vi "SetPWMFreq.vi"(8 "error in (no error)":errorcluster, 10 "Freq":sgl, 11 "PCA in":refnum<class "PCA.lvclass">) -> (0 "error out":errorcluster, 3 "PCA out":refnum<class "PCA.lvclass">)   [LabVIEW 2022 SP3, in "PCA9685.lvlib" / "PCA.lvclass"]
uses:
  PCA.lvclass
  PCA.lvclass/PCA.ctl
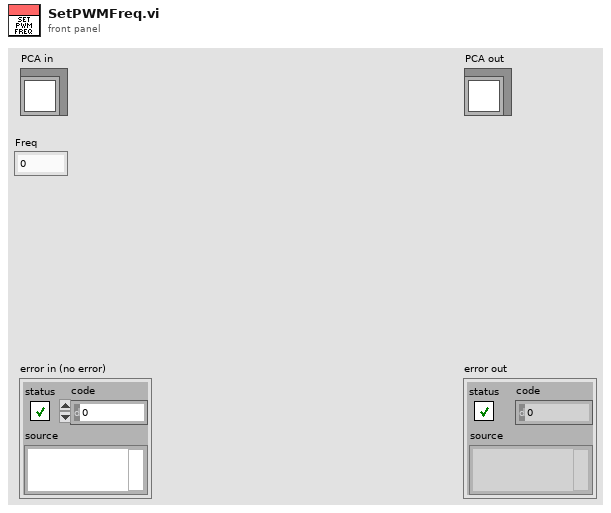
[diagram p1: front panel]
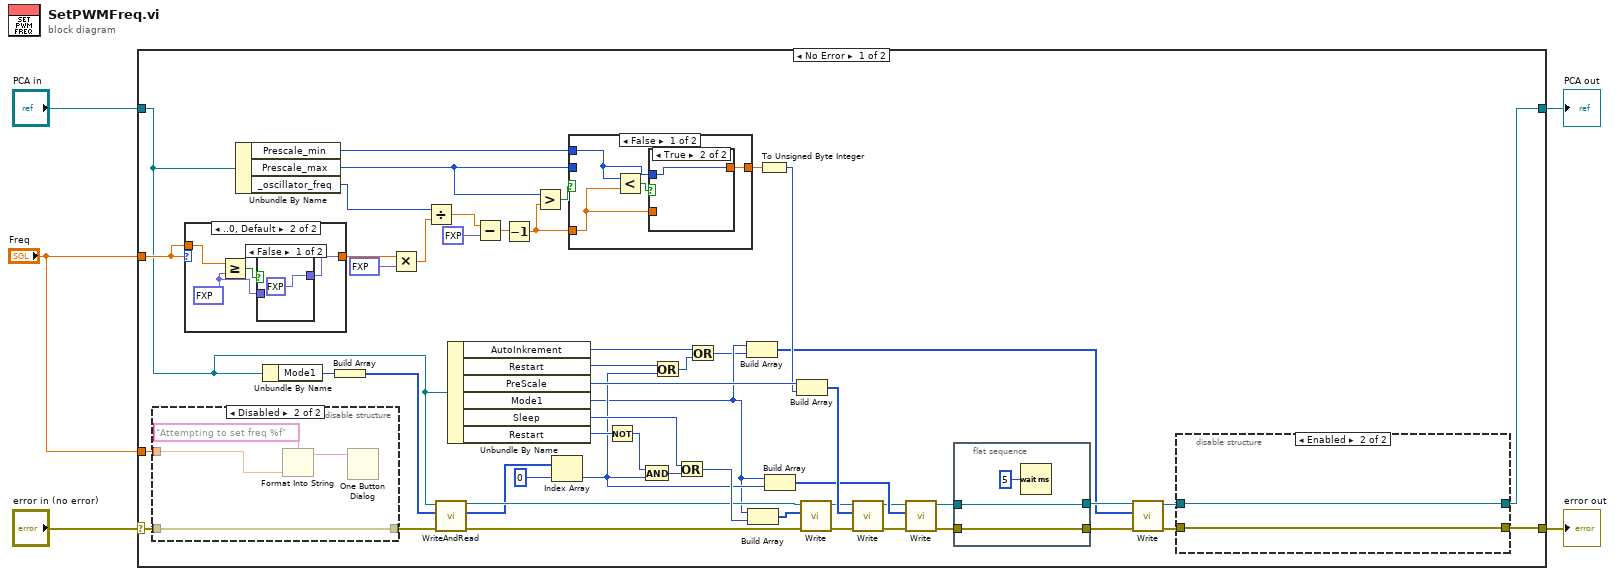
[diagram p0: block diagram]
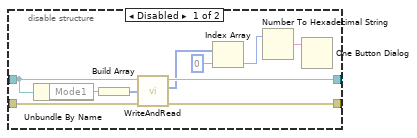
[diagram p2: hidden frame]
diagram:
  n1 = case shown="No Error" "error in (no error)" {
    selector: "error in (no error)" -> [w57 w93]
    tunnel: [w7 w93] -> w4
    tunnel: [w6 w92] -> w2
    tunnel: "PCA in" -> [w27 w92]
    tunnel: "Freq" -> [w56 _]
    tunnel: "Freq" -> [w55 _]
    frame No Error {
      n2 = disable-structure shown="Disabled" {
        disable-tunnel: w57 -> [w73 w77]
        disable-tunnel: [w73 w77] -> w54
        disable-tunnel: w56 -> [_ w76]
        frame Enabled {
        }
        frame Disabled {
          n3 = Format Into String(format string="Attempting to set freq %f", w76) -> (resulting string=w74:string)  [unwired: 2 in, 1 out]
          n4 = One Button Dialog(message=w74) -> ()  [unwired: 1 in, 1 out]
        }
      }
      n5 = case shown="..0, Default" w55 {
        tunnel: [w85 w89] -> w53
        tunnel: w55 -> [w85 w88]
        frame 1..3500 {
        }
        frame ..0, Default {
          w86 = fxp<+/-,64,32> 3500.0 ("y")
          n6 = Greater Or Equal?(x=w88, y=w86) -> (x >= y?=w87:bool)
          n7 = case shown="False" w87 {
            tunnel: [fxp<+/-,64,32> 1.0 ("Numeric") w91] -> w89
            tunnel: w86 -> [_ w91]
            frame False {
            }
            frame True {
            }
          }
        }
      }
      n8 = Unbundle By Name(w27) -> ("Prescale_min"=w43:u32, "Prescale_max"=w45:u32, "_oscillator_freq"=w50:u32)
      n9 = Unbundle By Name(w27) -> ("Mode1"=w42:u8)
      n10 = Build Array(w42) -> (w41:u8[])
      n11 = Multiply(x=w53, y=fxp<+/-,64,32> 4096.0) -> (x*y=w51:sgl)
      n12 = Divide(x=w50, y=w51) -> (x/y=w49:sgl)
      n13 = call "WriteAndRead.vi"("error in (no error)"=w54, "Data"=w41, "PCA in"=w27) -> ("error out"=w26:errorcluster, "Data 2"=w24:u8[], "PCA out"=w25:refnum<class "PCA.lvclass">)  [unwired: 6 in]
      n14 = Unbundle By Name(w27) -> ("AutoInkrement"=w16:u8, "Restart"=w18:u8, "PreScale"=w30:u8, "Mode1"=w11:u8, "Sleep"=w37:u8, "Restart"=w39:u8)
      n15 = Subtract(x=w49, y=fxp<+/-,64,33> 0.5) -> (x-y=w47:sgl)
      n16 = Decrement(x=w47) -> (x-1=w44:sgl)
      n17 = Greater?(x=w45, y=w44) -> (0:w46:bool)
      n18 = Index Array(array=w24, index=0) -> (element=w13:u8)
      n19 = case shown="False" w46 {
        tunnel: [w79 w84] -> w29
        tunnel: w45 -> [_ w84]
        tunnel: w44 -> [w78 _]
        tunnel: w43 -> [w80 _]
        frame False {
          n20 = Less?(x=w80, y=w78) -> (x < y?=w81:bool)
          n21 = case shown="True" w81 {
            tunnel: w80 -> [_ w83]
            tunnel: [w82 w83] -> w79
            tunnel: w78 -> [w82 _]
            frame False {
            }
            frame True {
            }
          }
        }
        frame True {
        }
      }
      n22 = Not(x=w39) -> (.not. x?=w38:u8)
      n23 = And(x=w38, y=w13) -> (x .and. y?=w40:u8)
      n24 = Or(x=w18, y=w13) -> (x .or. y?=w17:u8)
      n25 = Or(x=w37, y=w40) -> (x .or. y?=w35:u8)
      n26 = Or(x=w16, y=w17) -> (x .or. y?=w10:u8)
      n27 = Build Array(w11, w10) -> (w12:u8[])
      n28 = Build Array(w11, w35) -> (w34:u8[])
      n29 = To Unsigned Byte Integer(number=w29) -> (unsigned 8bit integer=w28:u8)
      n30 = Build Array(w11, w13) -> (w22:u8[])
      n31 = Build Array(w30, w28) -> (w33:u8[])
      n32 = call "Write.vi"("error in (no error)"=w26, "Data"=w34, "PCA in"=w25) -> ("error out"=w32:errorcluster, "PCA out"=w31:refnum<class "PCA.lvclass">)  [unwired: 7 in]
      n33 = call "Write.vi"("error in (no error)"=w32, "Data"=w33, "PCA in"=w31) -> ("error out"=w23:errorcluster, "PCA out"=w21:refnum<class "PCA.lvclass">)  [unwired: 7 in]
      n34 = call "Write.vi"("error in (no error)"=w23, "Data"=w22, "PCA in"=w21) -> ("error out"=w20:errorcluster, "PCA out"=w19:refnum<class "PCA.lvclass">)  [unwired: 7 in]
      n35 = flat-sequence {
        tunnel: w20 -> [w72]
        tunnel: [w72] -> w15
        tunnel: [w71] -> w14
        tunnel: w19 -> [w71]
        frame #0 {
          n36 = Wait (ms)(milliseconds to wait=u32 5) -> ()  [unwired: 1 out]
        }
      }
      n37 = call "Write.vi"("error in (no error)"=w15, "Data"=w12, "PCA in"=w14) -> ("error out"=w8:errorcluster, "PCA out"=w9:refnum<class "PCA.lvclass">)  [unwired: 7 in]
      n38 = disable-structure shown="Enabled" {
        disable-tunnel: w8 -> [w67 w68]
        disable-tunnel: w9 -> [w66 w69]
        disable-tunnel: [w63 w68] -> w7
        disable-tunnel: [w62 w69] -> w6
        frame Disabled {
          n39 = Unbundle By Name(w66) -> ("Mode1"=w65:u8)
          n40 = Build Array(w65) -> (w64:u8[])
          n41 = call "WriteAndRead.vi"("error in (no error)"=w67, "Data"=w64, "PCA in"=w66) -> ("error out"=w63:errorcluster, "Data 2"=w61:u8[], "PCA out"=w62:refnum<class "PCA.lvclass">)  [unwired: 6 in]
          n42 = Index Array(array=w61, index=0) -> (element=w59:u8)
          n43 = Number To Hexadecimal String(2:w59) -> (0:w58:string)  [unwired: 1 in]
          n44 = One Button Dialog(message=w58) -> ()  [unwired: 1 in, 1 out]
        }
        frame Enabled {
        }
      }
    }
    frame Error {
    }
  }
  "error out" <- w4
  "PCA out" <- w2
